vi "Setup Switch Device.vi"(11 "Instrument in":refnum<class "Instrument.lvclass">) -> (0 "error out":errorcluster)   [LabVIEW 2015, in "Instrument Close.lvclass"]
uses:
  Instrument Close.lvclass
  Classes/Instruments/Instrument/Class/Instrument.lvclass
  Classes/Instruments/Relay Control/Switch Executive/Switch Executive.lvclass
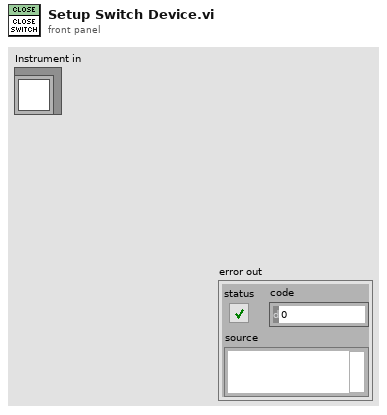
[diagram p1: front panel]
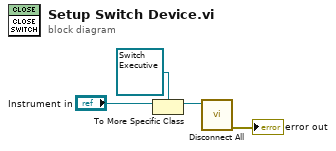
[diagram p0: block diagram]
diagram:
  n1 = To More Specific Class(target class=refnum<class "Switch Executive.lvclass"> refnum ("Switch Executive.lvlib:Switch Executive.lvclass"), reference="Instrument in") -> (specific class reference=w2:refnum<class "Switch Executive.lvclass">)  [unwired: 1 in, 1 out]
  n2 = call-dynamic "Disconnect All.vi"("Switch Executive in"=w2) -> ("error out"=→"error out":errorcluster)  [unwired: 9 in, 1 out]
